vi "get_speed_params.vi"(8 "error in (no error)":errorcluster, 11 "TrajectoryMG100122AODFrameScan in":refnum<class "TrajectoryMG100122AODFrameScan.lvclass">) -> (0 "error out":errorcluster, 1 "line-scan time":dbl[unit]=-1.0, 2 "frame rate":dbl[unit]=-1.0, 3 "TrajectoryMG100122AODFrameScan out":refnum<class "TrajectoryMG100122AODFrameScan.lvclass">, 4 "pixel-dwell time":dbl[unit]=-1e-06)   [LabVIEW 2010, in "TrajectoryMG100122AODFrameScan.lvclass"]
uses:
  TrajectoryMG100122AODFrameScan.lvclass
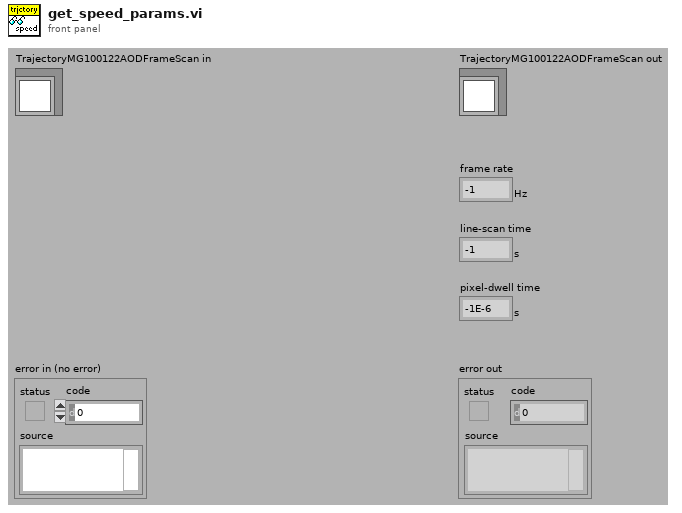
[diagram p1: front panel]
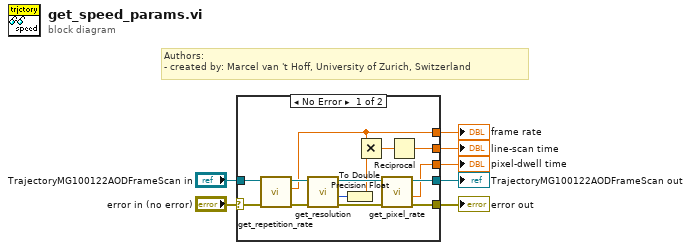
[diagram p0: block diagram]
diagram:
  # "Authors: \n- created by: Marcel van 't Hoff, University of Zurich, Switzerland"
  n1 = case shown="No Error" "error in (no error)" {
    selector: "error in (no error)" -> [w18 w23]
    tunnel: [w17 w23] -> w6
    tunnel: [w13 w22] -> w4
    tunnel: "TrajectoryMG100122AODFrameScan in" -> [w14 w22]
    tunnel: [w12 _] -> w3
    tunnel: [w9 _] -> w2
    tunnel: [w8 _] -> w1
    frame No Error {
      n2 = call-dynamic "get_repetition_rate.vi"("error in (no error)"=w18, "GenericTrajectory in"=w14) -> ("error out"=w20:errorcluster, "repetition rate"=w12:dbl[unit], "GenericTrajectory out"=w16:refnum<class "TrajectoryMG100122AODFrameScan.lvclass">)  [unwired: 7 in]
      n3 = call-dynamic "get_resolution.vi"("error in (no error)"=w20, "TrajectoryMG100122AODFrameScan in"=w16) -> ("error out"=w19:errorcluster, "y resolution"=w11:i32, "TrajectoryMG100122AODFrameScan out"=w15:refnum<class "TrajectoryMG100122AODFrameScan.lvclass">)  [unwired: 6 in, 1 out]
      n4 = To Double Precision Float(number=w11) -> (double precision float=w10:dbl)
      n5 = Multiply(x=w12, y=w10) -> (x*y=w21:dbl[unit])
      n6 = call-dynamic "get_pixel_rate.vi"("error in (no error)"=w19, "GenericTrajectory in"=w15) -> ("error out"=w17:errorcluster, "pixel dwell time"=w8:dbl[unit], "GenericTrajectory out"=w13:refnum<class "TrajectoryMG100122AODFrameScan.lvclass">)  [unwired: 6 in, 1 out]
      n7 = Reciprocal(x=w21) -> (1/x=w9:dbl[unit])
    }
    frame Error {
    }
  }
  "error out" <- w6
  "TrajectoryMG100122AODFrameScan out" <- w4
  "frame rate" <- w3
  "line-scan time" <- w2
  "pixel-dwell time" <- w1
